vi "testing.vi"() -> ()   [LabVIEW 2025]
uses:
  EnhancedWPI/JAS_CameraResolution.ctl
panel:
  in  "CameraResolution":T1
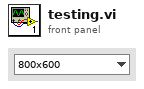
[diagram p1: front panel]
types:
  T1 = typedef "JAS_CameraResolution.ctl" = enum16{"800x600", "800x500", "800x450", "640x480", "640x400", "600x360", "320x256", "320x200", "320x180", "200x160", "200x125", "200x112", "160x128", "160x100", "160x90"}
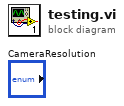
[diagram p0: block diagram]
diagram:
